vi "LVClass_CorrectionDataManager GetDiagnosticsEigenVector.vi"(0 "CorrectionDataManager in":refnum<class "CorrectionDataManager.lvclass">, 5 "n° mode":i32, 9 "HasoSlopes in":refnum<class "HasoSlopes.lvclass">, 11 "error in (no error)":errorcluster) -> (4 "CorrectionDataManager out":refnum<class "CorrectionDataManager.lvclass">, 8 "commands":sgl[](array[numeric]), 10 "HasoSlopes out":refnum<class "HasoSlopes.lvclass">, 15 "error out":errorcluster)   [LabVIEW 2020, in "CorrectionDataManager.lvclass"]
doc: "Get HasoSlopes object and commands array associated to an influence.\n\n--------------------------------------------------------------------------------\n\n<B>corrdata_managerIn </B> : CorrDataManager object.\n<B>corrdata_managerOut </B> : CorrDataManager object.\n<B>mode_index </B> : Influence index.\n<B>HasoSlopes </B> : HasoSlopes object.\n<B>commands </B> : Command array .\n<B>ErrorIn </B> : Error\n<B>ErrorOut </B> : Error\n\n--------------------------------------------------------------------------------"
uses:
  CorrectionDataManager.lvclass
  HasoSlopes.lvclass
  CorrectionDataManager.lvclass/CorrectionDataManager.ctl
  LVClass_HasoSlopes Read HasoSlopes _ property.vi
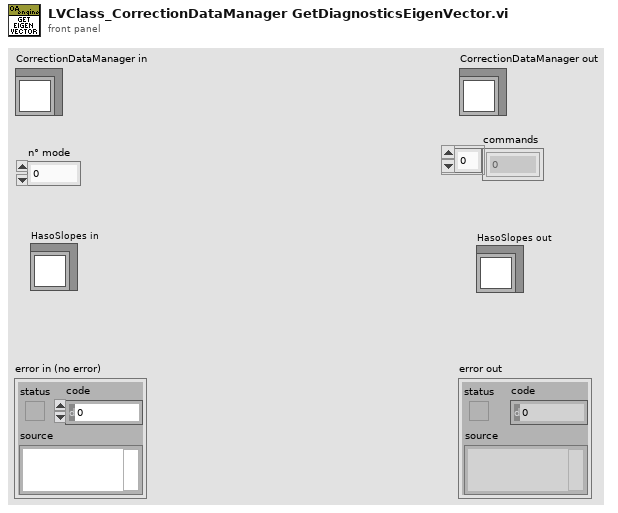
[diagram p1: front panel]
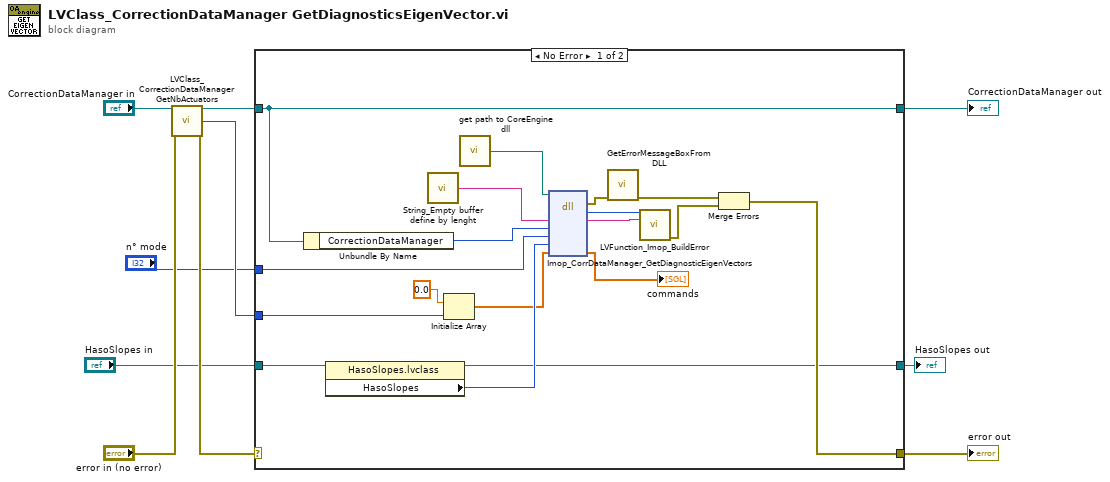
[diagram p0: block diagram]
diagram:
  n1 = call "LVClass_CorrectionDataManager GetNbActuators.vi"("CorrectionDataManager in"="CorrectionDataManager in", "error in (no error)"="error in (no error)") -> ("CorrectionDataManager out"=w7:refnum<class "CorrectionDataManager.lvclass">, "Nb actuators"=w6:i32, "error out"=w4:errorcluster)  [unwired: 11 in]
  n2 = case shown="No Error" w4 {
    selector: w4 -> [_ w31]
    tunnel: [w22 w31] -> w9
    tunnel: [w19 w30] -> w10
    tunnel: w7 -> [w19 w30]
    tunnel: w6 -> [w17 _]
    tunnel: "n° mode" -> [w16 _]
    tunnel: "HasoSlopes in" -> [w15 w29]
    tunnel: [w13 w29] -> w1
    frame No Error {
      n3 = Unbundle By Name(w19) -> ("CorrectionDataManager"=w18:i32)
      n4 = property class="HasoSlopes.lvclass"(reference=w15) -> (reference out=w13:refnum<class "HasoSlopes.lvclass">, "HasoSlopes"=w14:i32)  [unwired: 1 in, 1 out]
      n5 = call "String_Empty buffer define by lenght.vi"() -> ("Empty buffer"=w26:string)  [unwired: 1 in]
      n6 = Initialize Array(sgl 0.0, w17) -> (w12:sgl[])
      n7 = call "get path to CoreEngine dll.vi"() -> ("path to c_interface_vc100.dll"=w20:path)  [unwired: 12 in, 3 out]
      n8 = dll-call lib="D:/soft/HASO_v3/SVN_trunk/ImOpCoreEngine4_LV2011/DLLs/c_interface_vc100.dll" fn="Imop_CorrDataManager_GetDiagnosticEigenVectors"(path in=w20, "message"=w26, "corrdata_manager"=w18, "n° mode"=w16, "HasoSlopes"=w14, "commands"=w12) -> (error out=w25:errorcluster, "return type"=w28:i32, "message"=w27:string, "commands"=→"commands":sgl[])  [unwired: 5 in, 1 out]
      n9 = call "GetErrorMessageBoxFromDLL.vi"("error IN"=w25) -> ("error OUT"=w24:errorcluster)  [unwired: 10 in]
      n10 = call "LVFunction_Imop_BuildError.vi"("code"=w28, "String to Prepend to source (\"\")"=w27) -> ("error out"=w23:errorcluster)  [unwired: 13 in]
      n11 = Merge Errors(w24, w23) -> (w22:errorcluster)
    }
    frame Error {
    }
  }
  "error out" <- w9
  "CorrectionDataManager out" <- w10
  "HasoSlopes out" <- w1
